vi "PDW gen lfm for time.vi"(4 "center freqency":dbl=800000000.0 format="%#_13p", 5 "num of channels":i32, 6 "num of nano between channels":dbl, 7 "niqiest freqency":dbl=125000000.0 format="%#_13g", 8 "D.C":dbl=1.5 format="%#_13g", 9 "pulse amplitude":dbl format="%#_13g", 10 "pulse duration":dbl=0.1 format="%#_13g", 11 "frequency list":dbl[](array[numeric])=[60000000.0, 70000000.0, 130000000.0, 260000000.0]) -> (2 "niqiest band":dbl[](array[numeric])=[0.0, 1.0, 2.0], 3 "PDWs on channels":cluster{T1[]}[](array[cluster]))   [LabVIEW 2021]
uses:
  CTL/PDW_lv2.ctl
  CTL/mode_type.ctl
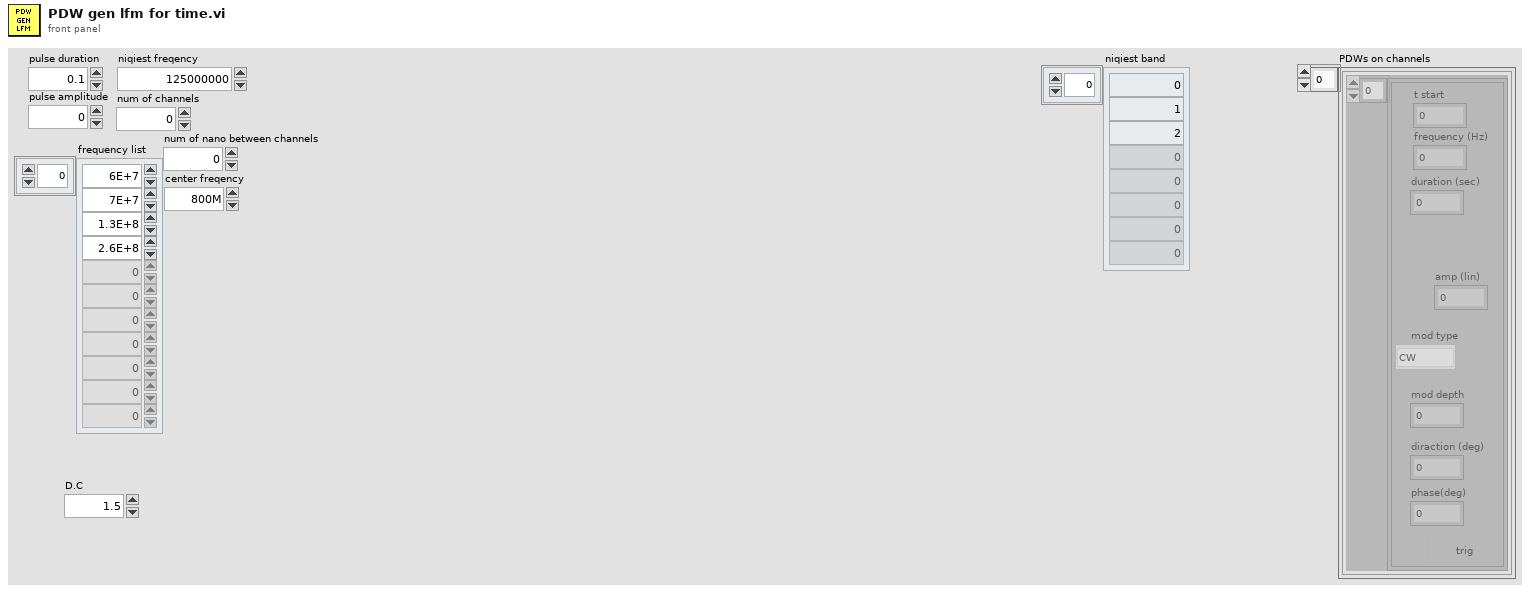
[diagram p1: front panel]
types:
  T1 = typedef "PDW_lv2.ctl" = cluster{"t start":dbl, "frequency (Hz)":dbl, "duration (sec)":dbl, "mod type":T2, "mod depth":dbl, "trig":bool, "amp (lin)":dbl, "diraction (deg)":dbl, "phase(deg)":dbl}
  T2 = typedef "mode_type.ctl" = enum8{"CW", "from memory 1", "NC - cw", "LFM", "BPSK", "QPSK"}
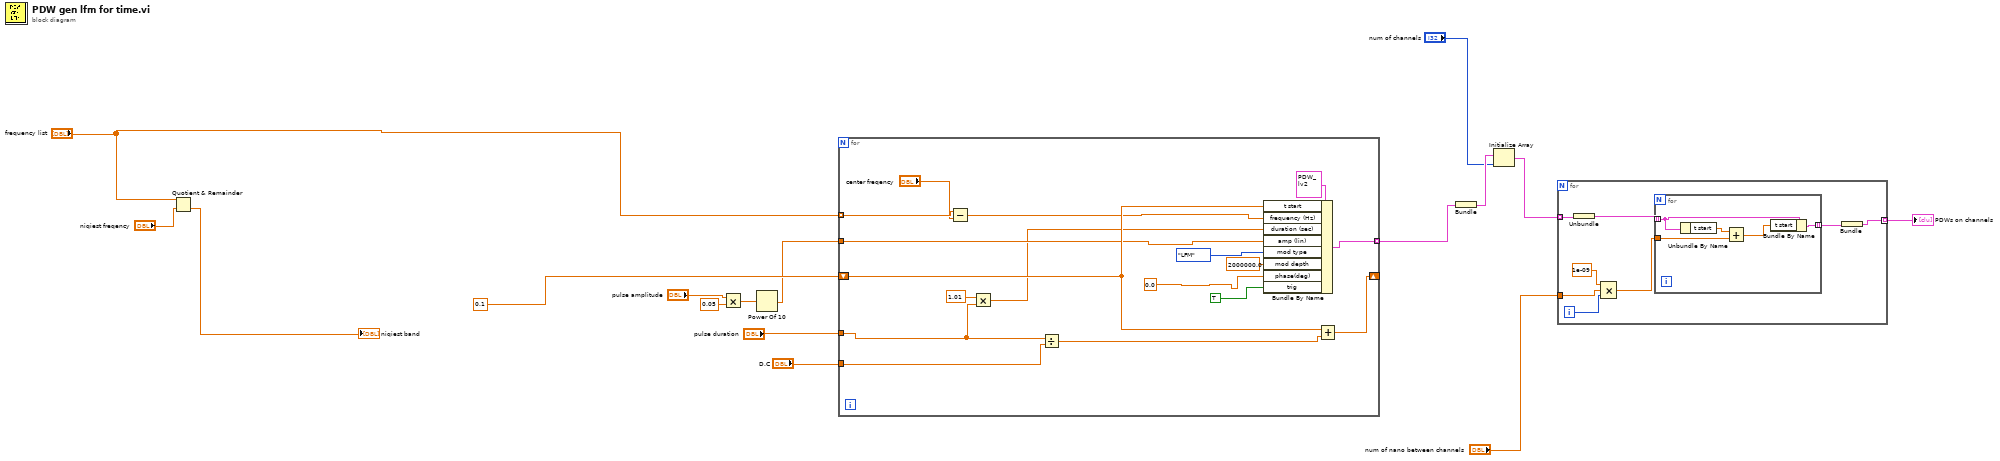
[diagram p0: block diagram]
diagram:
  n1 = Quotient & Remainder(x="frequency list", y="niqiest freqency") -> (floor(x/y)=→"niqiest band":dbl[])  [unwired: 1 out]
  n2 = Multiply(x="pulse amplitude", y=0.05) -> (x*y=w9:dbl)
  n3 = Power Of 10(x=w9) -> (10^x=w6:dbl)
  n4 = for {
    tunnel: "frequency list" -> [w30] mode=indexing
    tunnel: "pulse duration" -> [w26]
    shift-right: [w33] -> _
    shift-left: 0.1 -> [w31]
    tunnel: w6 -> [w28]
    tunnel: [w27] -> w14 mode=indexing
    tunnel: "D.C" -> [w23]
    n5 = Subtract(x=w30, y="center freqency") -> (x-y=w29:dbl)
    n6 = Multiply(x=1.01, y=w26) -> (x*y=w24:dbl)
    n7 = Divide(x=w26, y=w23) -> (x/y=w32:dbl)
    n8 = Bundle By Name(cluster=T1 {"t start"=0.0, "frequency (Hz)"=0.0, "duration (sec)"=0.0, "mod type"=enum."CW", "mod depth"=0.0, "trig"=FALSE, "amp (lin)"=0.0, "diraction (deg)"=0.0, "phase(deg)"=0.0}, "t start"=w31, "frequency (Hz)"=w29, "duration (sec)"=w24, "amp (lin)"=w28, "mod type"=mode_type."LFM", "mod depth"=2000000.0, "phase(deg)"=0.0 ("element"), "trig"=TRUE) -> (w27:T1)
    n9 = Add(x=w31, y=w32) -> (x+y=w33:dbl)
  }
  n10 = Bundle(w14) -> (w13:cluster{T1[]})  [unwired: 1 in]
  n11 = Initialize Array(w13, "num of channels") -> (w3:cluster{T1[]}[])
  n12 = for {
    tunnel: w3 -> [w41] mode=indexing
    tunnel: [w38] -> w2 mode=indexing
    tunnel: "num of nano between channels" -> [w36]
    i -> [w37]
    n13 = Unbundle(w41) -> (w40:T1[])
    n14 = Compound Arithmetic op=MULTIPLY(1e-09 ("x"), w36, w37) -> (w34:dbl)
    n15 = for {
      tunnel: w40 -> [w45] mode=indexing
      tunnel: [w43] -> w39 mode=indexing
      tunnel: w34 -> [w42]
      n16 = Unbundle By Name(w45) -> ("t start"=w46:dbl)
      n17 = Add(x=w46, y=w42) -> (x+y=w44:dbl)
      n18 = Bundle By Name(cluster=w45, "t start"=w44) -> (w43:T1)
    }
    n19 = Bundle(w39) -> (w38:cluster{T1[]})  [unwired: 1 in]
  }
  "PDWs on channels" <- w2
